vi "字符键盘.vi"(10 "显示样式":u32, 11 "原值":string) -> (3 "x+y":string)   [LabVIEW 2016, in "斯坦道CODMn.lvlib"]
uses:
  <vilib>/event_ctls.llb/eventvkey.ctl
panel:
  in  "M":bool
  in  "N":bool
  in  "B":bool
  in  "V":bool
  in  "C":bool
  in  "X":bool
  in  "Z":bool
  in  "L":bool
  in  "K":bool
  in  "J":bool
  in  "H":bool
  in  "G":bool
  in  "F":bool
  in  "D":bool
  in  "S":bool
  in  "A":bool
  in  "P":bool
  in  "O":bool
  in  "I":bool
  in  "U":bool
  in  "Y":bool
  in  "T":bool
  in  "R":bool
  in  "E":bool
  in  "W":bool
  in  "Q":bool
  in  "清除":bool
  in  "退格":bool
  in  "取消按钮":bool
  in  ".":bool
  out "字符串":string
  in  "0":bool
  in  "停止":bool
  in  "9":bool
  in  "8":bool
  in  "7":bool
  in  "6":bool
  in  "5":bool
  in  "4":bool
  in  "3":bool
  in  "2":bool
  in  "1":bool
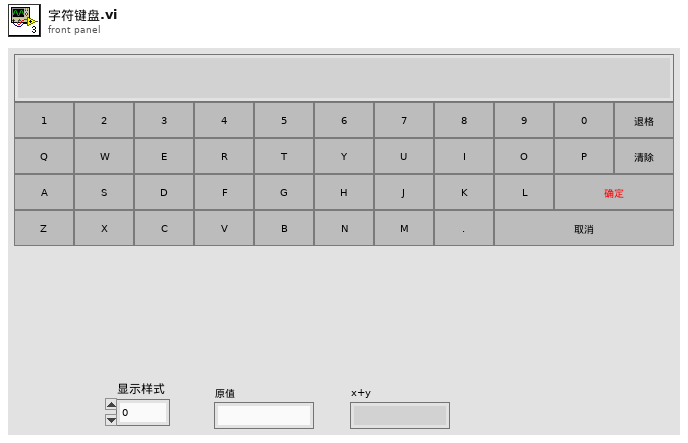
[diagram p1: front panel]
types:
  T1 = typedef "eventvkey.ctl" = enum16{"ASCII", "Enter", "Return", "Shift", "Ctrl", "Alt", "Cmd", "Opt", "Caps", "NumLock", "Clear", "Break", "Up", "Down", "Left", "Right", "Insert", "Delete", "Home", "End", "PageUp", "PageDown", "Escape", "Help", "Pause", "ScrollLock", "F1", "F2", "F3", "F4", "F5", "F6", "F7", "F8", "F9", "F10", "F11", "F12", "F13", "F14", "F15", "F16", "F17", "F18", "F19", "F20", "F21", "F22", "F23", "F24", "Play", "VolumeUp", "VolumeDown", "Mute", "Two Byte Char"}
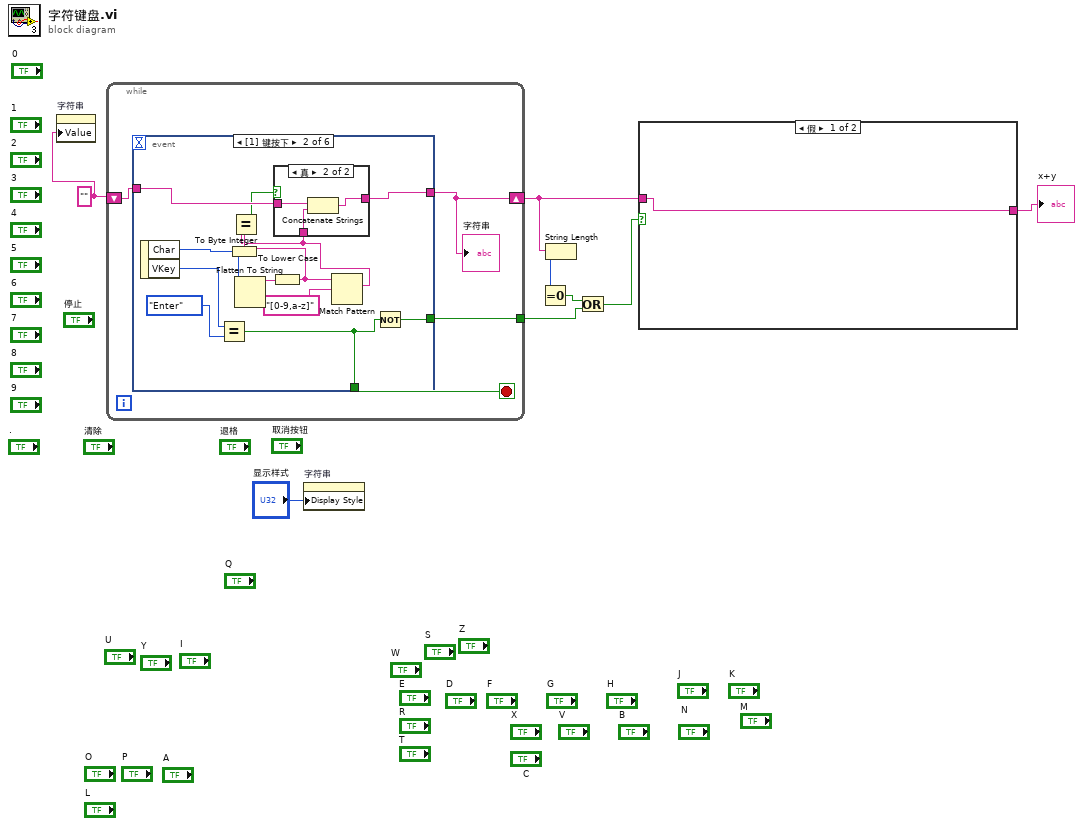
[diagram p0: block diagram]
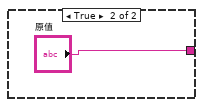
[diagram p2: hidden frame]
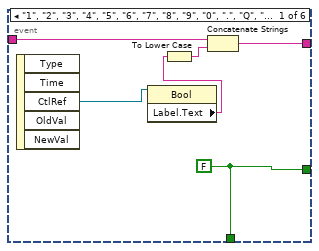
[diagram p3: hidden frame]
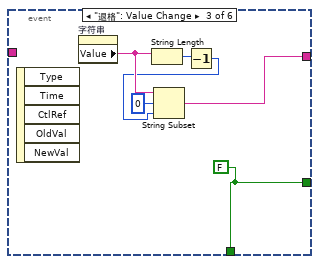
[diagram p5: hidden frame]
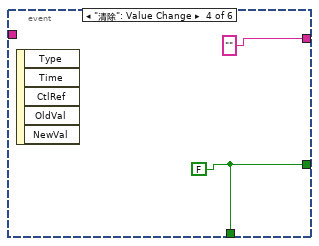
[diagram p6: hidden frame]
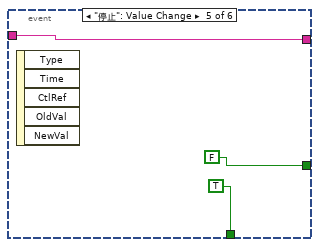
[diagram p7: hidden frame]
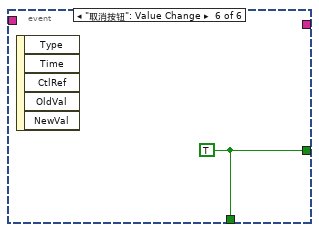
[diagram p8: hidden frame]
diagram:
  w8 = "" ("Label.Text")
  n1 = property on="字符串" class="Str"("Value"=w8) -> ()  [unwired: 2 in, 2 out]
  n2 = while {
    shift-right: [w11] -> w7
    shift-left: w8 -> [w10]
    tunnel: [w9] -> w2
    stop <- w12 stop-if-true
    n3 = event shown="[1] 键按下" {
      selector: _ -> [_ _ _ _ _ _]
      dyn-events: _ -> [_ _ _ _ _ _]
      timeout: _ -> [_ _ _ _ _ _]
      tunnel: [w15 w20 w36 w42 TRUE w47] -> w12
      tunnel: [w17 w28 w37 "" ("Label.Text") w45 _] -> w11
      tunnel: w10 -> [w16 w27 _ _ w45 _]
      tunnel: [w15 w21 w36 w42 FALSE w47] -> w9
      event "1", "2", "3", "4", "5", "6", "7", "8", "9", "0", ".", "Q", "W", "E", "R", "T", "Y", "U", "I", "O", "P", "A", "S", "D", "F", "G", "H", "J", "K", "L", "Z", "X", "C", "V", "B", "N", "M": Value Change {
        w15 = FALSE
        n4 = event-data() -> ("CtlRef"=w18:refnum<vi>)  [unwired: 1 in, 4 out]
        n5 = property class="Bool"(reference=w18) -> ("Label.Text"=w13:string)  [unwired: 1 in, 2 out]
        n6 = To Lower Case(string=w13) -> (all lower case string=w14:string)
        n7 = Concatenate Strings(w16, w14) -> (w17:string)
      }
      event Key Down {
        n8 = event-data() -> ("Char"=w31:i16, "VKey"=w19:T1)  [unwired: 1 in]
        n9 = Equal?(x=w19, y=eventvkey."Enter" ("V键")) -> (x = y?=w20:bool)
        n10 = To Byte Integer(number=w31) -> (8bit integer=w30:i8)
        n11 = Flatten To String(anything=w30) -> (data string=w29:string)  [unwired: 3 in, 2 out]
        n12 = To Lower Case(string=w29) -> (all lower case string=w25:string)
        n13 = Match Pattern(string=w25, regular expression="[0-9,a-z]" ("正则表达式")) -> (match substring=w24:string)  [unwired: 1 in, 3 out]
        n14 = Equal?(x=w25, y=w24) -> (x = y?=w23:bool)
        n15 = case shown="真" w23 {
          tunnel: [w32 w35] -> w28
          tunnel: w27 -> [w32 w34]
          tunnel: w24 -> [_ w33]
          frame False {
          }
          frame True {
            n16 = Concatenate Strings(w34, w33) -> (w35:string)
          }
        }
        n17 = Not(x=w20) -> (.not. x?=w21:bool)
      }
      event "退格": Value Change {
        w36 = FALSE
        n18 = event-data() -> ()  [unwired: 1 in, 5 out]
        n19 = property on="字符串" class="Str"() -> ("Value"=w40:string)  [unwired: 2 in, 2 out]
        n20 = String Length(string=w40) -> (length=w41:i32)
        n21 = Decrement(x=w41) -> (x-1=w38:i32)
        n22 = String Subset(string=w40, offset (0)=0 ("偏移量(0)"), length (rest)=w38) -> (substring=w37:string)
      }
      event "清除": Value Change {
        w42 = FALSE
        n23 = event-data() -> ()  [unwired: 1 in, 5 out]
      }
      event "停止": Value Change {
        n24 = event-data() -> ()  [unwired: 1 in, 5 out]
      }
      event "取消按钮": Value Change {
        w47 = TRUE
        n25 = event-data() -> ()  [unwired: 1 in, 5 out]
      }
    }
    "字符串" <- w11
  }
  n26 = property on="字符串" class="Str"("Display Style"="显示样式") -> ()  [unwired: 2 in, 2 out]
  n27 = String Length(string=w7) -> (length=w6:i32)
  n28 = Equal To 0?(x=w6) -> (x = 0?=w5:bool)
  n29 = Or(x=w5, y=w2) -> (x .or. y?=w4:bool)
  n30 = case shown="假" w4 {
    tunnel: w7 -> [w48 _]
    tunnel: [w48 "原值"] -> w3
    frame False {
    }
    frame True {
    }
  }
  "x+y" <- w3
